vi "GetNumHiSpeedDevices.vi"(3 "error in (no error)":errorcluster) -> (0 "error out":errorcluster, 1 "device count":u32, 2 "result":u32)   [LabVIEW 2010]
uses:
  FTCSPI.dll
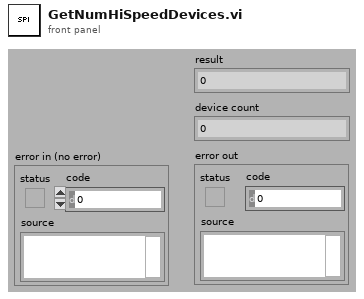
[diagram p1: front panel]
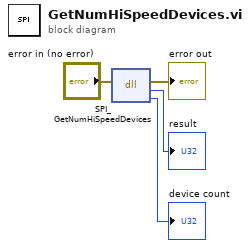
[diagram p0: block diagram]
diagram:
  n1 = dll-call lib="C:/Users/Administrator/Documents/GitHub/labview/FPGA/FTCSPI.dll" fn="SPI_GetNumHiSpeedDevices"(error in="error in (no error)") -> (error out=→"error out":errorcluster, "result"=→"result":u32, "device count"=→"device count":u32)  [unwired: 3 in, 1 out]
